vi "Query Class.vi"(7 "Selection Info":T1, 8 "error in":errorcluster, 11 "LVClassLibrary Refnum":refnum<vi>) -> (0 "error out":errorcluster, 3 "Class Info":T1, 4 "Class Locked?":bool)   [LabVIEW 2020, in "ConstantErrorsMaker.lvlib"]
uses:
  ConstantErrorsMaker.lvlib
  Selection Info--cluster.ctl
  Selection Type--enum.ctl
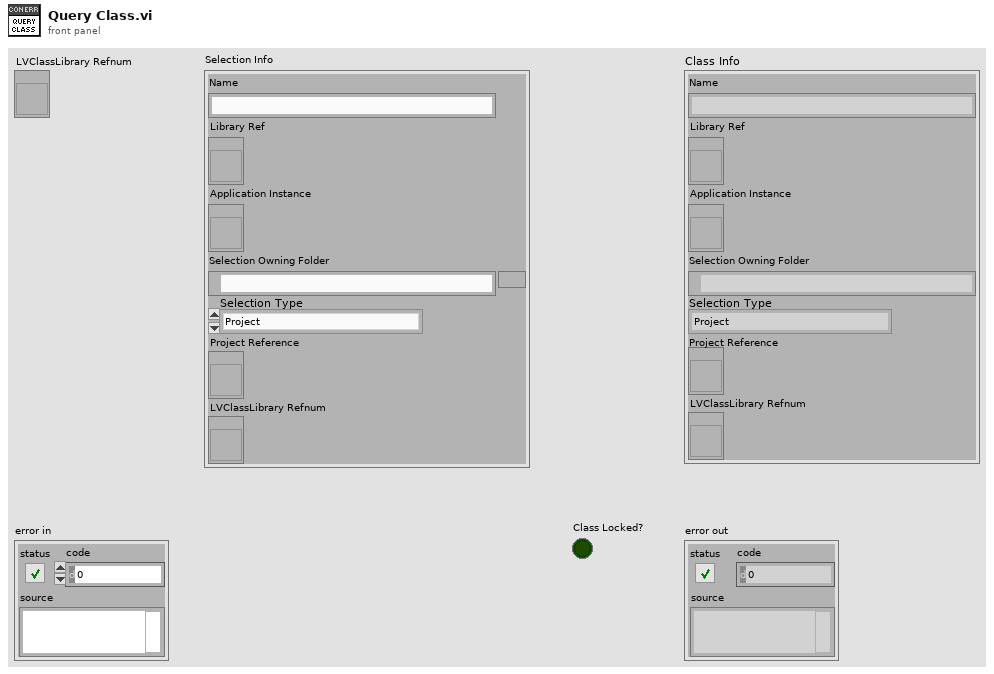
[diagram p1: front panel]
types:
  T1 = typedef "ConstantErrorsMaker.lvlib/Selection Info--cluster.ctl" = cluster{"Name":string, "Library Ref":refnum<vi>, "Application Instance":refnum<vi>, "Selection Owning Folder":path, "Selection Type":T2, "Project Reference":refnum<vi>, "LVClassLibrary Refnum":refnum<vi>}
  T2 = typedef "ConstantErrorsMaker.lvlib/Selection Type--enum.ctl" = enum16{"Project", "Library", "Class", "DQMH Singleton", "DQMH Cloneable"}
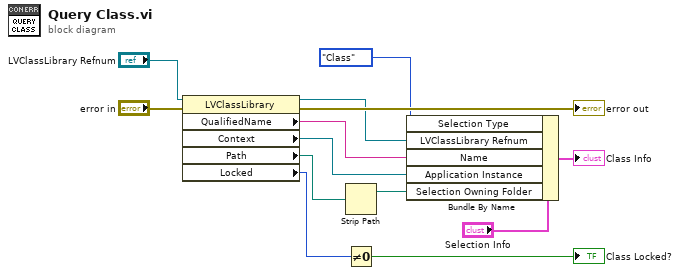
[diagram p0: block diagram]
diagram:
  n1 = property class="LVClassLibrary"(reference="LVClassLibrary Refnum", error in="error in") -> (reference out=w2:refnum<vi>, error out=→"error out":errorcluster, "QualifiedName"=w11:string, "Context"=w8:refnum<vi>, "Path"=w10:path, "Locked"=w6:i32)
  n2 = Strip Path(path=w10) -> (stripped path=w9:path)  [unwired: 1 out]
  n3 = Not Equal To 0?(x=w6) -> (x != 0?=→"Class Locked?":bool)
  n4 = Bundle By Name(cluster="Selection Info", "Selection Type"=Selection_Type--enum."Class", "LVClassLibrary Refnum"=w2, "Name"=w11, "Application Instance"=w8, "Selection Owning Folder"=w9) -> (→"Class Info":T1)
